vi "InitDrv_thread.vi"(8 "error in (no error)":errorcluster) -> (0 "error out":errorcluster)   [LabVIEW 2015, in "ESLSCDLL.lvlib"]
uses:
  ESLSCDLL.lvlib
  Globals.vi
  ESLSCDLL.dll
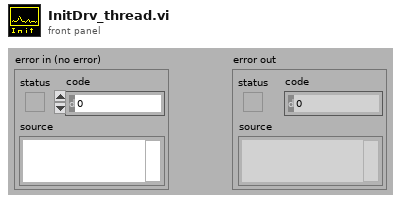
[diagram p1: front panel]
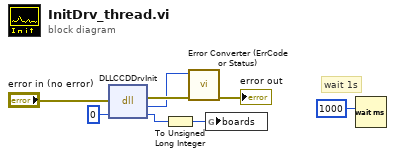
[diagram p0: block diagram]
diagram:
  # "wait 1s"
  n1 = dll-call lib="C:/ENTW/PCIE/LV64/board.vis/ESLSCDLL.dll" fn="DLLCCDDrvInit"(error in="error in (no error)", "number_of_boards"=u8 0) -> (error out=w6:errorcluster, "es_status_codes"=w5:i32, "number_of_boards"=w3:u8)  [unwired: 2 in, 1 out]
  n2 = To Unsigned Long Integer(number=w3) -> (unsigned 32bit integer=w2:u32)
  n3 = call "Error Converter (ErrCode or Status).vi"("error in (no error)"=w6, "error code"=w5) -> ("error out"=→"error out":errorcluster)  [unwired: 9 in]
  n4 = global write "Globals.vi" "boards"(w2) -> ()
  n5 = Wait (ms)(milliseconds to wait=u32 1000) -> ()  [unwired: 1 out]
